vi "trigger parent vi.vi"(11 "T=continuous, F=finite":bool) -> (0 "error out":errorcluster, 3 "ctr tasks out":refnum<k21>[](array[refnum]))   [LabVIEW 2012]
doc: "SciScan 1.2 160622"
uses:
  GFG/GFGnumericGet.vi
  GFG/GFGbooleanGet.vi
  GFG/GFG library.lvlib
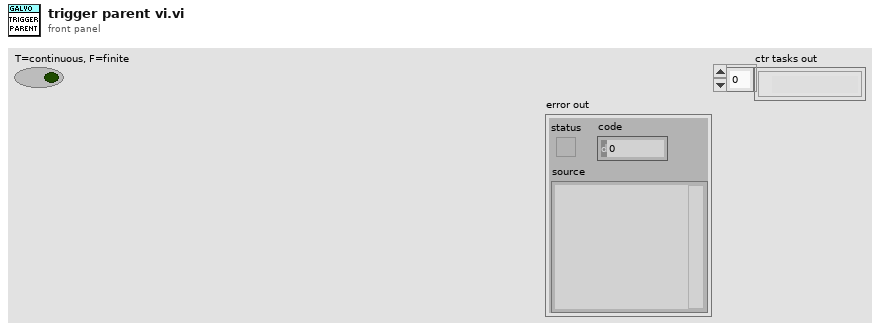
[diagram p1: front panel]
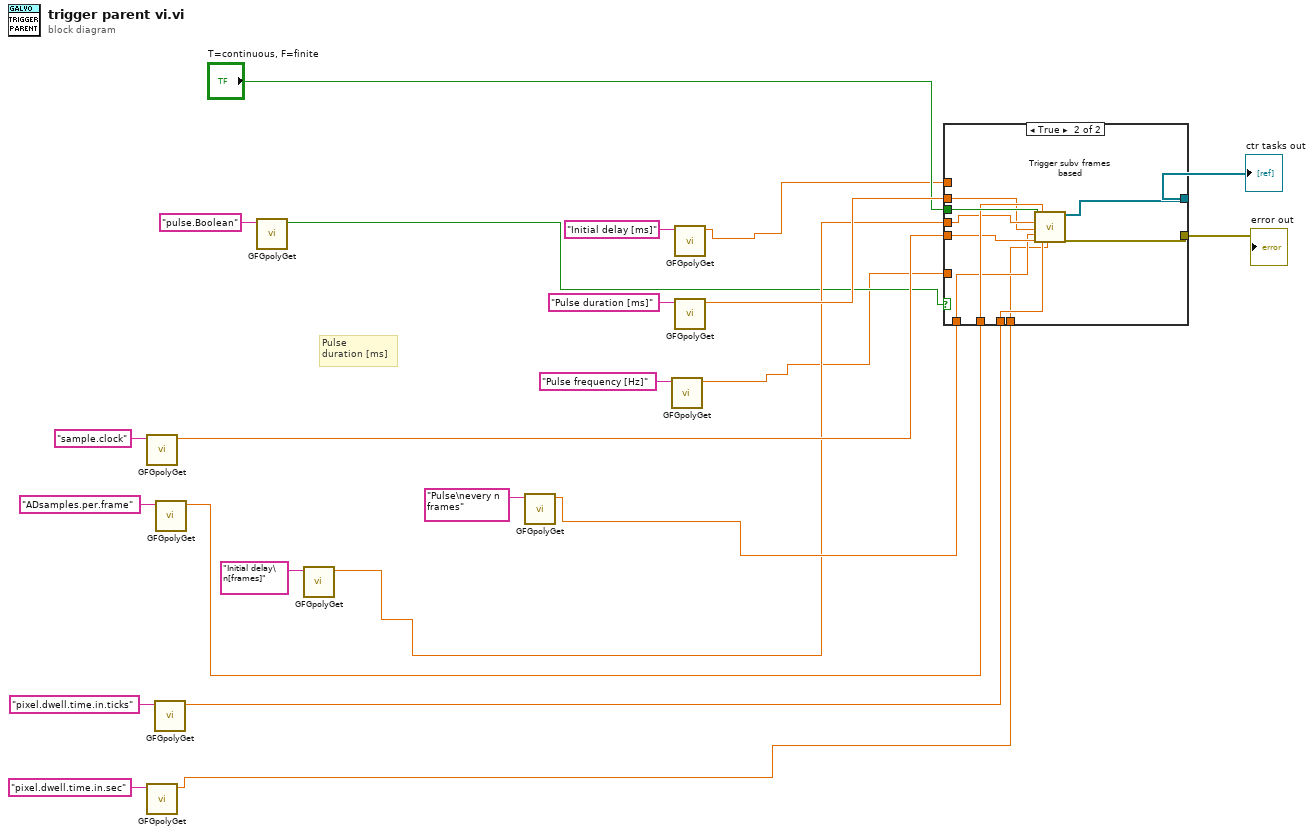
[diagram p0: block diagram]
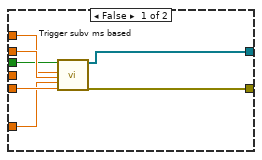
[diagram p2: hidden frame]
diagram:
  # "Pulse\nduration [ms]"
  n1 = call-poly "GFGpolyGet.vi"("Variable Name in"="sample.clock") -> ("Numeric"=w13:dbl)  [unwired: 8 in, 2 out]
  n2 = call-poly "GFGpolyGet.vi"("Variable Name in"="pixel.dwell.time.in.sec") -> ("Numeric"=w7:dbl)  [unwired: 8 in, 2 out]
  n3 = call-poly "GFGpolyGet.vi"("Variable Name in"="pixel.dwell.time.in.ticks") -> ("Numeric"=w1:dbl)  [unwired: 8 in, 2 out]
  n4 = call-poly "GFGpolyGet.vi"("Variable Name in"="ADsamples.per.frame") -> ("Numeric"=w3:dbl)  [unwired: 8 in, 2 out]
  n5 = call-poly "GFGpolyGet.vi"("Variable Name in"="pulse.Boolean") -> ("Boolean Value OUT"=w4:bool)  [unwired: 9 in, 1 out]
  n6 = call-poly "GFGpolyGet.vi"("Variable Name in"="Initial delay\n[frames]") -> ("Numeric"=w5:dbl)  [unwired: 8 in, 2 out]
  n7 = call-poly "GFGpolyGet.vi"("Variable Name in"="Pulse\nevery n frames") -> ("Numeric"=w6:dbl)  [unwired: 8 in, 2 out]
  n8 = call-poly "GFGpolyGet.vi"("Variable Name in"="Pulse frequency [Hz]") -> ("Numeric"=w2:dbl)  [unwired: 8 in, 2 out]
  n9 = call-poly "GFGpolyGet.vi"("Variable Name in"="Initial delay [ms]") -> ("Numeric"=w10:dbl)  [unwired: 8 in, 2 out]
  n10 = call-poly "GFGpolyGet.vi"("Variable Name in"="Pulse duration [ms]") -> ("Numeric"=w21:dbl)  [unwired: 8 in, 2 out]
  n11 = case shown="True" w4 {
    tunnel: w21 -> [w30 w31]
    tunnel: "T=continuous, F=finite" -> [w29 w38]
    tunnel: [w28 w39] -> w17
    tunnel: [w27 w40] -> w16
    tunnel: w13 -> [w26 w35]
    tunnel: w10 -> [w25 _]
    tunnel: w2 -> [w24 _]
    tunnel: w3 -> [_ w37]
    tunnel: w1 -> [_ w36]
    tunnel: w7 -> [_ w32]
    tunnel: w6 -> [_ w34]
    tunnel: w5 -> [_ w33]
    frame False {
      n12 = call "Trigger subv ms based.vi"("T=continuous, F=finite"=w29, "Initial delay [ms]"=w25, "Pulse duration [ms]"=w30, "Pulse frequency [Hz]"=w24, "Sample clock rate"=w26) -> ("ctr tasks out"=w27:refnum<k21>[], "error out"=w28:errorcluster)  [unwired: 13 in]
    }
    frame True {
      n13 = call "Trigger subv frames based.vi"("T=continuous, F=finite"=w38, "Initial delay\n[frames]"=w33, "Pulse duration [ms]"=w31, "Pulse\nevery n frames"=w34, "Sample clock rate"=w35, "ADsamples.per.frame"=w37, "pixel.dwell.time.in.ticks"=w36, "pixel.dwell.time.in.sec"=w32) -> ("ctr tasks out"=w40:refnum<k21>[], "error out"=w39:errorcluster)  [unwired: 10 in]
    }
  }
  "error out" <- w17
  "ctr tasks out" <- w16
